vi "move direction V1.2.vi"(2 "theta":dbl, 3 "offset":dbl format="%#_13g") -> (0 "max value":dbl, 1 "out array":dbl[](array[numeric]))   [LabVIEW 2019]
panel:
  out "appended array":dbl[](array[numeric])
  out "theta 2":dbl
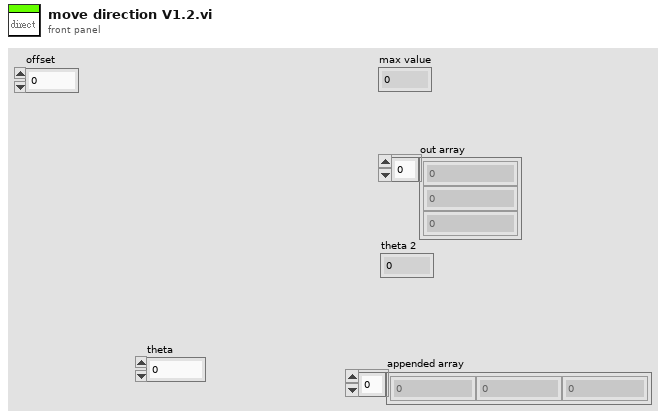
[diagram p1: front panel]
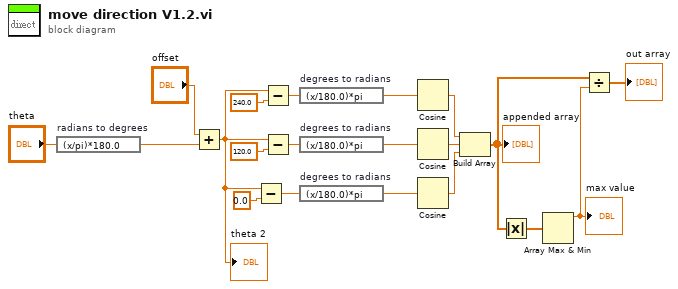
[diagram p0: block diagram]
diagram:
  n1 = expression code="(x/pi)*180.0" "radians to degrees"("theta") -> (w3:dbl)
  n2 = Add(x="offset", y=w3) -> (x+y=w2:dbl)
  "theta 2" <- w2
  n3 = Subtract(x=w2, y=0.0) -> (x-y=w11:dbl)
  n4 = Subtract(x=w2, y=240.0) -> (x-y=w13:dbl)
  n5 = Subtract(x=w2, y=120.0) -> (x-y=w12:dbl)
  n6 = expression code="(x/180.0)*pi" "degrees to radians"(w13) -> (w10:dbl)
  n7 = expression code="(x/180.0)*pi" "degrees to radians"(w12) -> (w9:dbl)
  n8 = expression code="(x/180.0)*pi" "degrees to radians"(w11) -> (w8:dbl)
  n9 = Cosine(x=w10) -> (cos(x)=w17:dbl)
  n10 = Cosine(x=w9) -> (cos(x)=w19:dbl)
  n11 = Cosine(x=w8) -> (cos(x)=w18:dbl)
  n12 = Build Array(w17, w19, w18) -> (w5:dbl[])
  "appended array" <- w5
  n13 = Absolute Value(x=w5) -> (abs(x)=w6:dbl[])
  n14 = Array Max & Min(array=w6) -> (max value=w4:dbl)  [unwired: 3 out]
  "max value" <- w4
  n15 = Divide(x=w5, y=w4) -> (x/y=→"out array":dbl[])
